vi "open.vi"(8 "error in (no error)":errorcluster, 10 "Path":path, 11 "ScriptEditorV2 in":refnum<class "ScriptEditorV2.lvclass">) -> (0 "error out":errorcluster, 3 "ScriptEditorV2 out":refnum<class "ScriptEditorV2.lvclass">)   [LabVIEW 2011, in "Views.lvlib" / "ScriptEditor.lvlib" / "ScriptEditorV2.lvclass"]
uses:
  ScriptEditorV2.lvclass
  Tools/Scripting/DataPointScript/DataPointScript.lvclass
  ScriptEditorV2.lvclass/ScriptEditorV2.ctl
  Tools/Scripting/ScriptingEvent/ScriptEventList/ScriptEventList.lvclass
  Tools/DatabaseHelpers/DbConnection/DeviceDataBase/deviceDataBase.lvclass
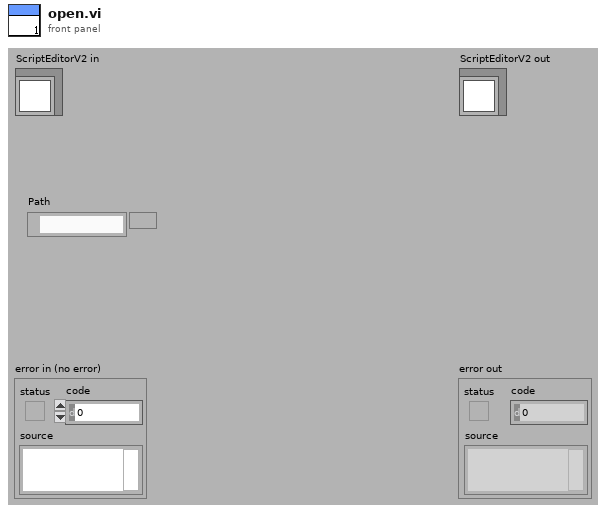
[diagram p1: front panel]
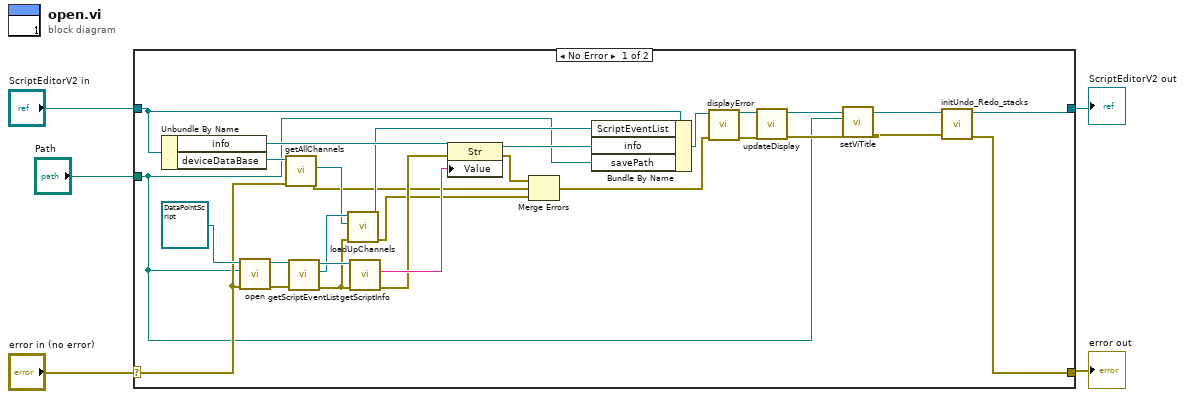
[diagram p0: block diagram]
diagram:
  n1 = case shown="No Error" "error in (no error)" {
    selector: "error in (no error)" -> [w21 w36]
    tunnel: [w6 w36] -> w4
    tunnel: [w7 w35] -> w1
    tunnel: "ScriptEditorV2 in" -> [w24 w35]
    tunnel: "Path" -> [w10 _]
    frame No Error {
      n2 = Unbundle By Name(w24) -> ("info"=w30:refnum<vi>, "deviceDataBase"=w22:refnum<class "deviceDataBase.lvclass">)
      n3 = call "open.vi"("error in (no error)"=w21, "Path"=w10, "DataPointScript in"=refnum<class "DataPointScript.lvclass"> refnum ("Tools.lvlib:Scripting.lvlib:DataPointScript.lvclass")) -> ("error out"=w32:errorcluster, "DataPointScript out"=w33:refnum<class "DataPointScript.lvclass">)  [unwired: 7 in]
      n4 = call "getAllChannels.vi"("error in (no error)"=w21, "deviceDataBase in"=w22) -> ("error out"=w19:errorcluster, "ChannelArray.lvclass"=w20:refnum<class "ChannelArray.lvclass">)  [unwired: 7 in, 1 out]
      n5 = call "getScriptEventList.vi"("error in (no error)"=w32, "DataPointScript.lvclass in"=w33) -> ("error out"=w23:errorcluster, "ScriptEventList"=w26:refnum<class "ScriptEventList.lvclass">, "DataPointScript.lvclass out"=w31:refnum<class "DataPointScript.lvclass">)  [unwired: 7 in]
      n6 = call "loadUpChannels.vi"("error in (no error)"=w23, "ChannelArray"=w20, "ScriptEventList in"=w26) -> ("error out"=w18:errorcluster, "ScriptEventList out"=w25:refnum<class "ScriptEventList.lvclass">)  [unwired: 7 in]
      n7 = call "getScriptInfo.vi"("error in (no error)"=w23, "DataPointScript.lvclass in"=w31) -> ("error out"=w28:errorcluster, "Script info"=w29:string)  [unwired: 7 in, 1 out]
      n8 = property class="Str"(reference=w30, error in=w28, "Value"=w29) -> (reference out=w27:refnum<vi>, error out=w17:errorcluster)
      n9 = Merge Errors(w17, w19, w18) -> (w15:errorcluster)
      n10 = Bundle By Name(cluster=w24, "ScriptEventList"=w25, "info"=w27, "savePath"=w10) -> (w16:refnum<class "ScriptEditorV2.lvclass">)
      n11 = call "displayError.vi"("error in (no error)"=w15, "ScriptEditorV2 in"=w16) -> ("error out"=w13:errorcluster, "ScriptEditorV2 out"=w14:refnum<class "ScriptEditorV2.lvclass">)  [unwired: 8 in]
      n12 = call "updateDisplay.vi"("error in (no error)"=w13, "ScriptEditorV2 in"=w14) -> ("error out"=w11:errorcluster, "ScriptEditorV2 out"=w12:refnum<class "ScriptEditorV2.lvclass">)  [unwired: 8 in]
      n13 = call "setViTitle.vi"("error in (no error)"=w11, "Path"=w10, "ScriptEditorV2 in"=w12) -> ("error out"=w8:errorcluster, "ScriptEditorV2 out"=w9:refnum<class "ScriptEditorV2.lvclass">)  [unwired: 7 in]
      n14 = call "initUndo_Redo_stacks.vi"("error in (no error)"=w8, "ScriptEditorV2 in"=w9) -> ("error out"=w6:errorcluster, "ScriptEditorV2 out"=w7:refnum<class "ScriptEditorV2.lvclass">)  [unwired: 8 in]
    }
    frame Error {
    }
  }
  "error out" <- w4
  "ScriptEditorV2 out" <- w1
